vi "ClienteTCP_17_05_envio_a_micro (1) (1).vi"() -> ()   [LabVIEW 2020]
uses:
  <vilib>/Instr/_visa.llb/VISA Configure Serial Port (Instr).vi
  <vilib>/addons/control/pid/pid.llb/PID (DBL).vi
  <vilib>/addons/control/pid/NI_PID_pid.lvlib
  <vilib>/ptbypt/NI_PtbyPt.lvlib
panel:
  out "PWM":dbl(graph)
  out "Error de Iluminacion":u32(graph)
  out "Ref vs Iluminacion":cluster{u32, "lux (decimal)":u32}(graph)
  out "output":dbl format="%.2f"
  in  "PID gains":T1={"proportional gain (Kc)"=1.0, "integral time (Ti, min)"=0.01, "derivative time (Td, min)"=0.0} {"derivative time (Td, min)" format="%.3f"; "integral time (Ti, min)" format="%.3f"; "proportional gain (Kc)" format="%.3f"}
  in  "output range":cluster{"output high":dbl, "output low":dbl}={"output high"=100.0, "output low"=-100.0} {"output low" format="%.2f"; "output high" format="%.2f"}
  in  "Referencia de iluminación":dbl(knob) scale=0.0..6000.0
  in  "VISA resource name":refnum<visa-resource-name>
  out "lux (decimal)":u32
  out "x = y?":bool
  out "longitud_restante":i32
  out "Valor lux":string
  in  "mode (standard)":T2(ring)
  out "data out":string
  in  "bytes to read":i32
  in  "stop":bool
  in  "puerto":u16
  in  "address":string
  # "CLIENTE"
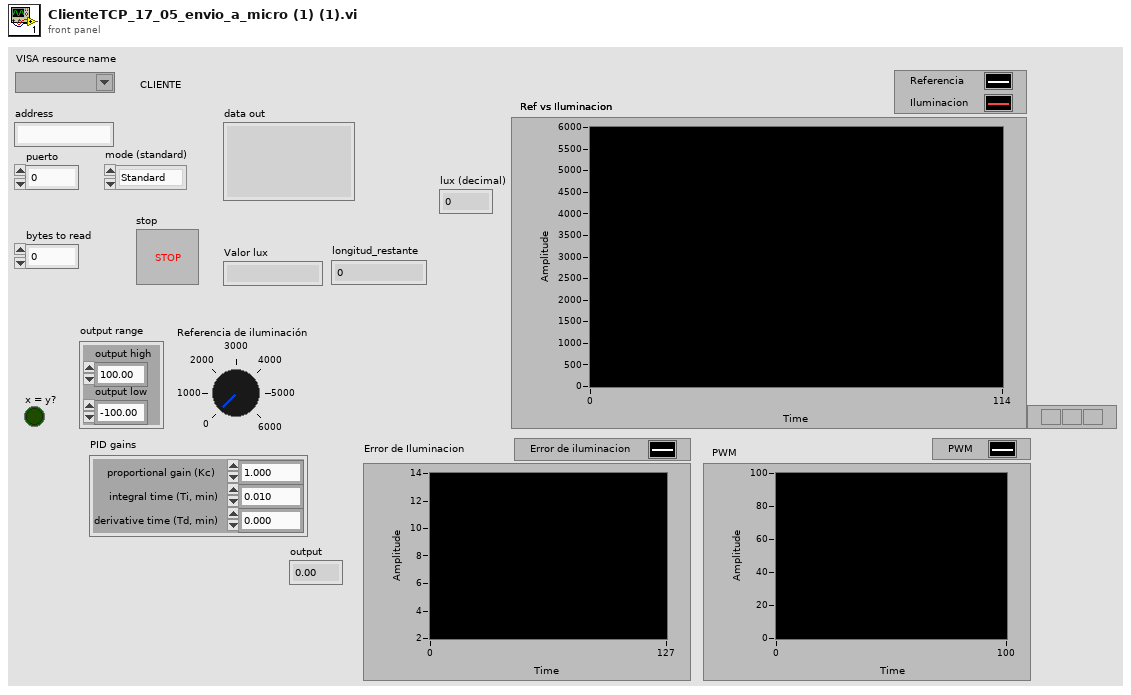
[diagram p1: front panel]
types:
  T1 = cluster{"proportional gain (Kc)":dbl, "integral time (Ti, min)":dbl, "derivative time (Td, min)":dbl}
  T2 = enum16{"Standard", "Buffered", "CRLF", "Immediate"}
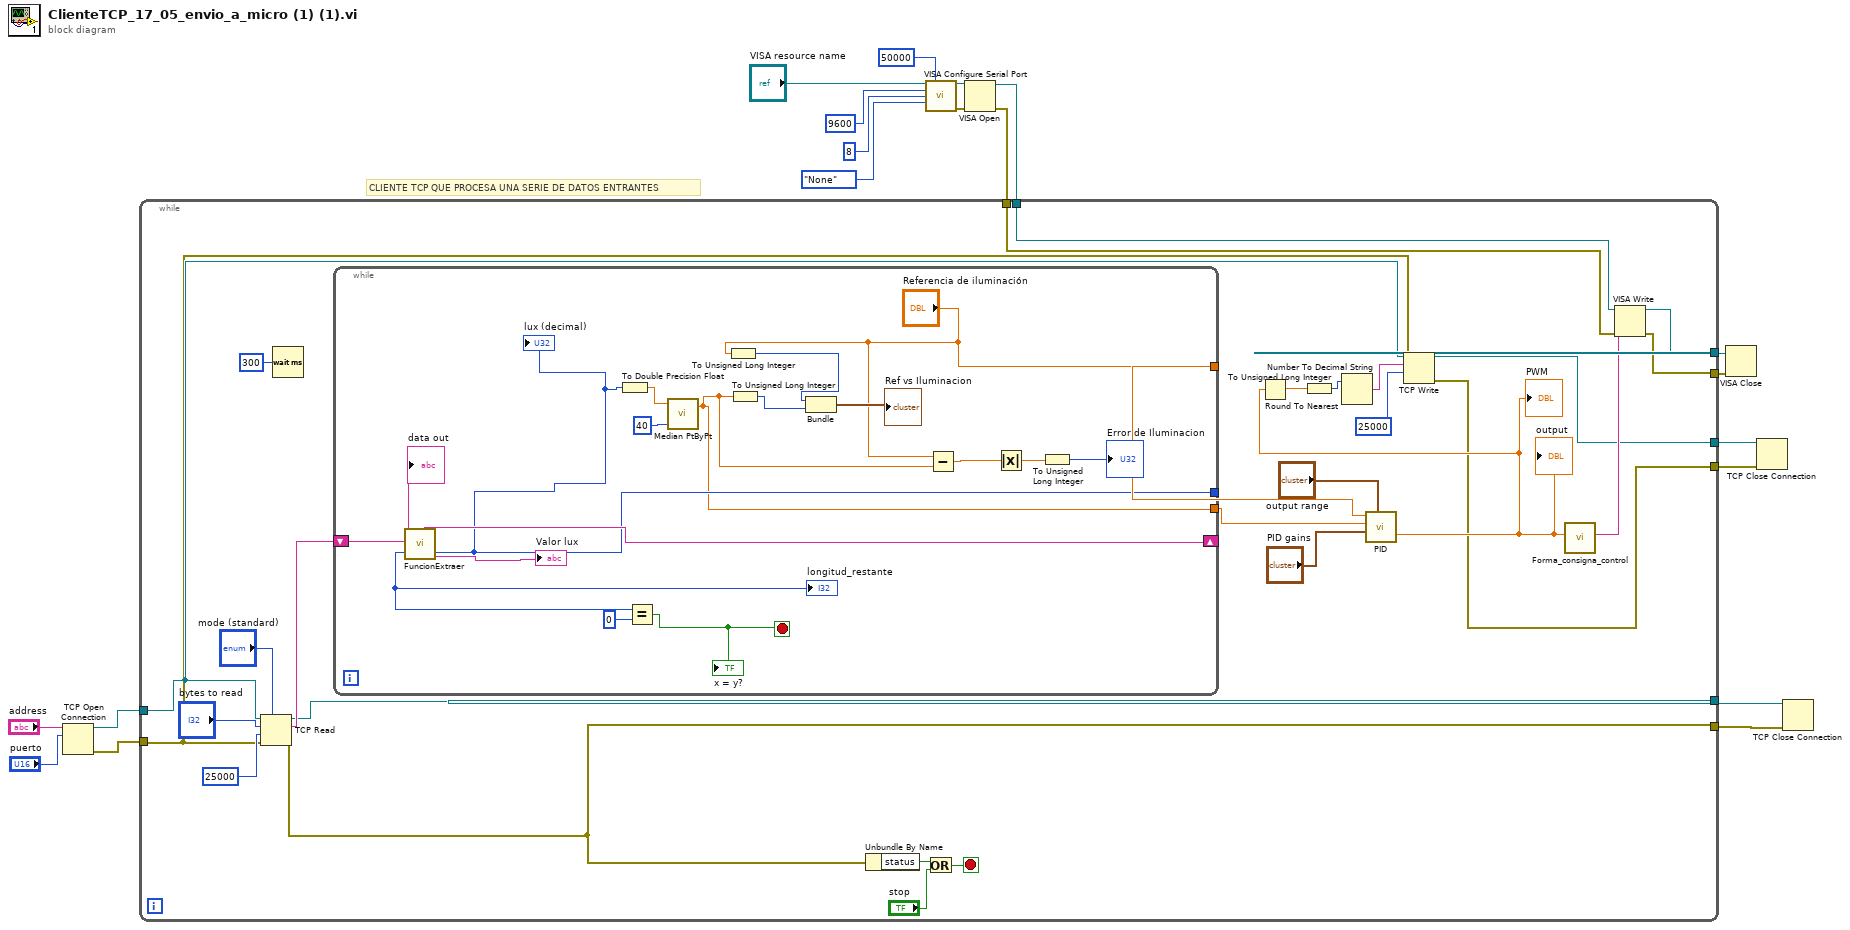
[diagram p0: block diagram]
diagram:
  # "CLIENTE TCP QUE PROCESA UNA SERIE DE DATOS ENTRANTES"
  n1 = TCP Open Connection(address="address", remote port or service name="puerto") -> (connection ID=w17:refnum<k5>, error out=w15:errorcluster)  [unwired: 3 in]
  n2 = call-poly "VISA Configure Serial Port"("VISA resource name"="VISA resource name", "timeout (10sec)"=u32 50000, "baud rate (9600)"=u32 9600, "data bits (8)"=u16 8, "parity (0:none)"=enum16{"None", "Odd", "Even", "Mark", "Space"}."None") -> ("VISA resource name out"=w9:refnum<visa-resource-name>, "error out"=w8:errorcluster)  [unwired: 9 in]
  n3 = VISA Open(error in (no error)=w8, VISA resource name=w9) -> (VISA resource name=w6:refnum<visa-resource-name>, error out=w5:errorcluster)  [unwired: 3 in]
  n4 = while {
    tunnel: w17 -> [w21]
    tunnel: [w28] -> w16
    tunnel: w15 -> [w20]
    tunnel: [w26] -> w14
    tunnel: w6 -> [w38]
    tunnel: w5 -> [w39]
    tunnel: [w36] -> w4
    tunnel: [w37] -> w3
    tunnel: [w27] -> w2
    tunnel: [w25] -> w1
    stop <- w45 stop-if-true
    n5 = TCP Read(connection ID=w21, bytes to read="bytes to read", error in (no error)=w20, 7:"mode (standard)", 9:25000 ("timeout ms (25000)")) -> (connection ID out=w28:refnum<k5>, data out=w41:string, error out=w26:errorcluster)
    n6 = Wait (ms)(milliseconds to wait=u32 300) -> ()  [unwired: 1 out]
    n7 = while {
      shift-right: [w64] -> _
      shift-left: w41 -> [w59]
      tunnel: [w55] -> _
      tunnel: ["Referencia de iluminación"] -> w32
      tunnel: [w51] -> w31
      stop <- w60 stop-if-true
      n8 = call "FuncionExtraer.vi"("Buffer entrada"=w59) -> ("Valor lux"=→"Valor lux":string, "lux (decimal)"=w55:u32, "after substring"=w64:string, "longitud_restante"=w61:i32)  [unwired: 6 in, 1 out]
      "longitud_restante" <- w61
      "lux (decimal)" <- w55
      n9 = To Double Precision Float(number=w55) -> (double precision float=w56:dbl)
      n10 = Equal?(x=w61, y=0) -> (x = y?=w60:bool)
      "x = y?" <- w60
      n11 = call <vilib>:"Median PtByPt.vi"("sample length"=40, "x"=w56) -> ("median"=w51:dbl)  [unwired: 2 in, 1 out]
      n12 = To Unsigned Long Integer(number="Referencia de iluminación") -> (unsigned 32bit integer=w58:u32)
      n13 = To Unsigned Long Integer(number=w51) -> (unsigned 32bit integer=w53:u32)
      n14 = Bundle(w58, w53) -> (→"Ref vs Iluminacion":cluster{u32, u32})  [unwired: 1 in]
      n15 = Subtract(x="Referencia de iluminación", y=w51) -> (x-y=w50:dbl)
      n16 = Absolute Value(x=w50) -> (abs(x)=w49:dbl)
      n17 = To Unsigned Long Integer(number=w49) -> (unsigned 32bit integer=→"Error de Iluminacion":u32)
      "data out" <- w59
    }
    n18 = Unbundle By Name(w26) -> ("status"=w47:bool)
    n19 = Or(x=w47, y="stop") -> (x .or. y?=w45:bool)
    n20 = call-poly <vilib>:"PID.vi"("output range"="output range", "PID gains"="PID gains", "process variable"=w31, "setpoint"=w32) -> ("output"=w29:dbl)  [unwired: 6 in, 1 out]
    "output" <- w29
    "PWM" <- w29
    n21 = Round To Nearest(number=w29) -> (nearest integer value=w30:dbl)
    n22 = To Unsigned Long Integer(number=w30) -> (unsigned 32bit integer=w23:u32)
    n23 = Number To Decimal String(number=w23) -> (decimal integer string=w22:string)  [unwired: 1 in]
    n24 = TCP Write(connection ID=w21, data in=w22, error in (no error)=w20, 9:25000 ("timeout ms (25000)")) -> (connection ID out=w27:refnum<k5>, error out=w25:errorcluster)  [unwired: 1 out]
    n25 = call "Forma_consigna_control.vi"("number"=w29) -> ("concatenated string"=w33:string)  [unwired: 10 in]
    n26 = VISA Write(VISA resource name=w38, write buffer=w33, error in (no error)=w39) -> (VISA resource name out=w36:refnum<visa-resource-name>, error out=w37:errorcluster)  [unwired: 1 out]
  }
  n27 = VISA Close(VISA resource name=w4, error in (no error)=w3) -> ()  [unwired: 1 out]
  n28 = TCP Close Connection(connection ID=w2, error in (no error)=w1) -> ()  [unwired: 1 in, 2 out]
  n29 = TCP Close Connection(connection ID=w16, error in (no error)=w14) -> ()  [unwired: 1 in, 2 out]
